vi "PowerGenerated.vi"() -> ()   [LabVIEW 2019]
uses:
  SubVis/Location.ctl
  <vilib>/Analysis/baseanly.llb/Mean (DBL).vi
  <vilib>/Utility/file.llb/Read Delimited Spreadsheet (DBL).vi
  <vilib>/Analysis/NI_AALBase.lvlib
panel:
  out "Day of Max Power":i32 caption="Day:"
  out "Max Power":dbl caption="Max Power:" format="%#_3pW"
  in  "Location":T1
  out "Max Power (watts)":dbl(slide) caption="2.1MW" scale=0.0..40000000.0 scale format="%#_6pW"
  in  "Stop":bool
  in  "USA":bool
  in  "CostaRica":bool
  in  "Brazil":bool
  in  "India":bool
  in  "Australia":bool
  in  "Japan":bool
  in  "SouthAfrica":bool
  in  "Israel":bool
  in  "Germany":bool
  in  "Days of Month":u8(slide)=30 min=1 max=30 step=1 scale=1.0..30.0
  out "USA_Select":u16(ring)
  out "Germany_Select":u16(ring)
  out "Brazil_Select":u16(ring)
  out "Israel_Select":u16(ring)
  out "India_Select":u16(ring)
  out "Japan_Select":u16(ring)
  out "SouthAfrica_Select":u16(ring)
  out "Australia_Select":u16(ring)
  out "CostaRica_Select":u16(ring)
  out "Wind Speed of All Countries":waveform(dbl)[](graph)
  out "Power Per Country":dbl[](graph)
  # "The day of maximum power output for a given location is determined for all days starting from the first day of the month until the selected day. The power output and corresponding day are displayed numerically and the power output is also displayed on a meter."
  # "Choose the location and day of the month that you would like to be displayed on the Power Per Country graph. All data from the first day of the month up until the selected day will be displayed."
  # "All countries wind speed data over 30 days is displayed on this graph."
  # "TO DO:  \nWind plot gets thicker when country is selected.\nTips slide down from above in semitransparent window."
  # "40MW"
  # "MAX POWER:"
  # "Move the mouse over included countried to see a plot of their power generation capabilities.  The windspeed for the selected county is highlighted in the graph at the lower right.  \n\nThe  Max Power can be viewed in the top right indicator and graphically on the meter at the far right.  The peak Day appears as a dotted line.\n\nThe slide control above selects how many days in the month are viewed."
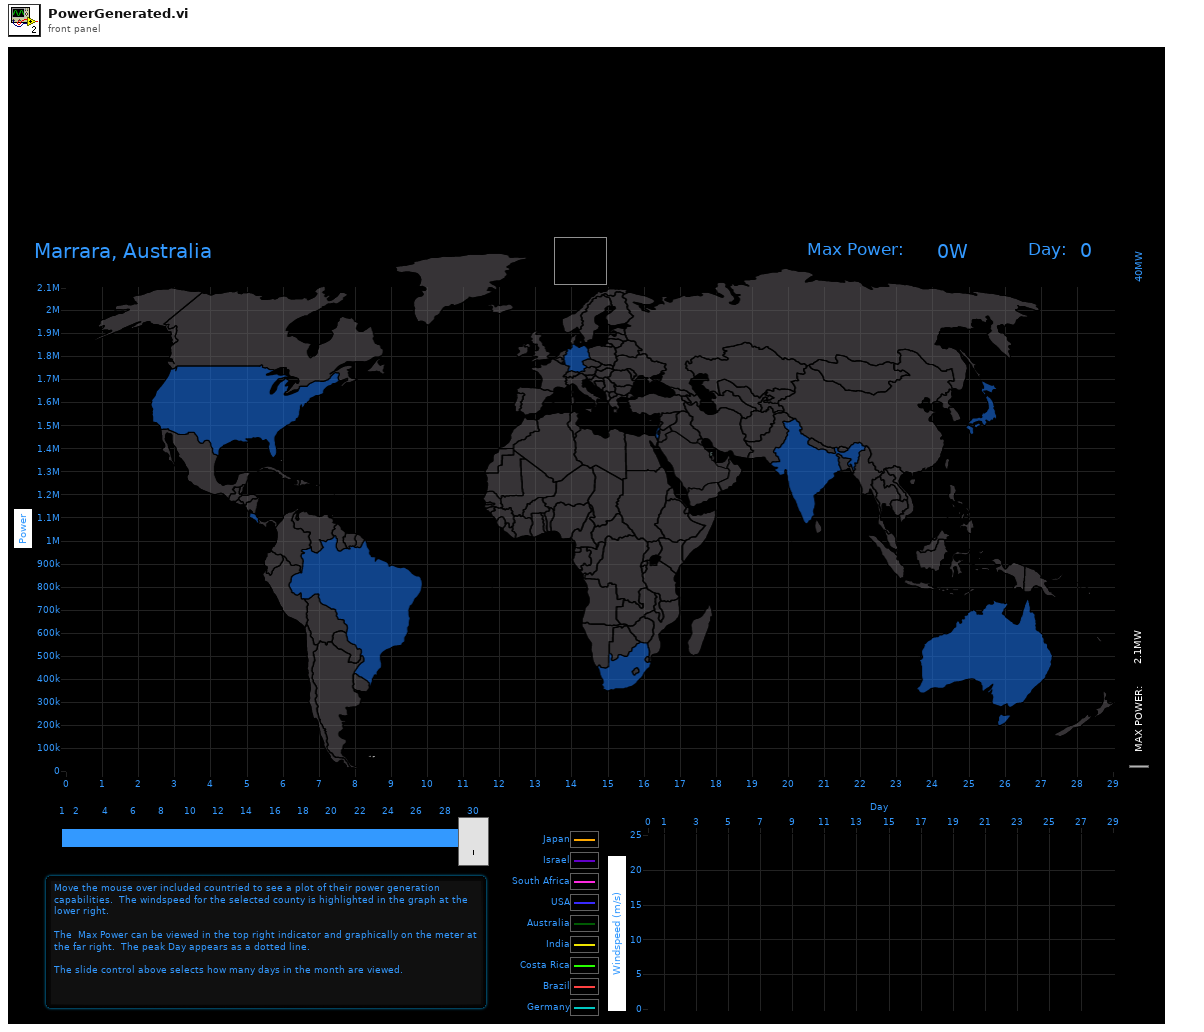
[diagram p1: front panel]
types:
  T1 = typedef "Location.ctl" = enum16{"Marrara, Australia", "Brasilia, Brazil", "Puerto Limon, Costa Rica", "Berlin, Germany", "Mumbai, India", "Sde-Dov, Israel", "Ise Bay, Japan", "Cape Good Hope, South Africa", "Texas, USA"}
  T2 = enum32{"invalid app kind", "Development System", "Run Time System", "Student Edition", "Embedded LabVIEW", "Evaluation", "Custom"}
  T3 = cluster{"Name":string, "Color":u32, "Style":u8, "Point Style":u8, "Name Visible":bool, "Allow Drag":bool, "Cursor Mode":u32, "Plot":i32, "Index":i32, "Position":cluster{"X":i32, "Y":i32}, "X Scale":u32, "Y Scale":u32, "Watch Plots":i32[], "Watch All Plots":bool, "Plot Area":i32, "Label Offset":cluster{"X":dbl, "Y":dbl}}
  T4 = cluster{"Name":string, "Color":u32, "Style":u8, "Point Style":u8, "Name Visible":bool, "Allow Drag":bool, "Annotation Mode":u32, "Plot":i32, "Index":i32, "Position":cluster{"X":dbl, "Y":dbl}, "X Scale":u32, "Y Scale":u32, "Show Arrow":bool, "Lock Name":bool, "Plot Area":i32, "Label Offset":cluster{"X":dbl, "Y":dbl}}
  T5 = cluster{"Location":T1, "Max Power":dbl, "Days of Month":u8, "Power Per Country":dbl[], "Day of Max Power":i32}
  T6 = cluster{"Name":string, "Color":u32, "Style":u8, "Point Style":u8, "Name Visible":bool, "Allow Drag":bool, "Annotation Mode":u32, "Plot":i32, "Index":i32, "Position":cluster{"X":dbl, "Y":dbl}, "X Scale":u32, "Y Scale":u32, "Show Arrow":bool, "Lock Name":bool, "Plot Area":i32, "Label Offset":cluster{"X":dbl, "Y":dbl}}[]
  T7 = cluster{"Name":string, "Color":u32, "Style":u8, "Point Style":u8, "Name Visible":bool, "Allow Drag":bool, "Cursor Mode":u32, "Plot":i32, "Index":i32, "Position":cluster{"X":i32, "Y":i32}, "X Scale":u32, "Y Scale":u32, "Watch Plots":i32[], "Watch All Plots":bool, "Plot Area":i32, "Label Offset":cluster{"X":dbl, "Y":dbl}}[]
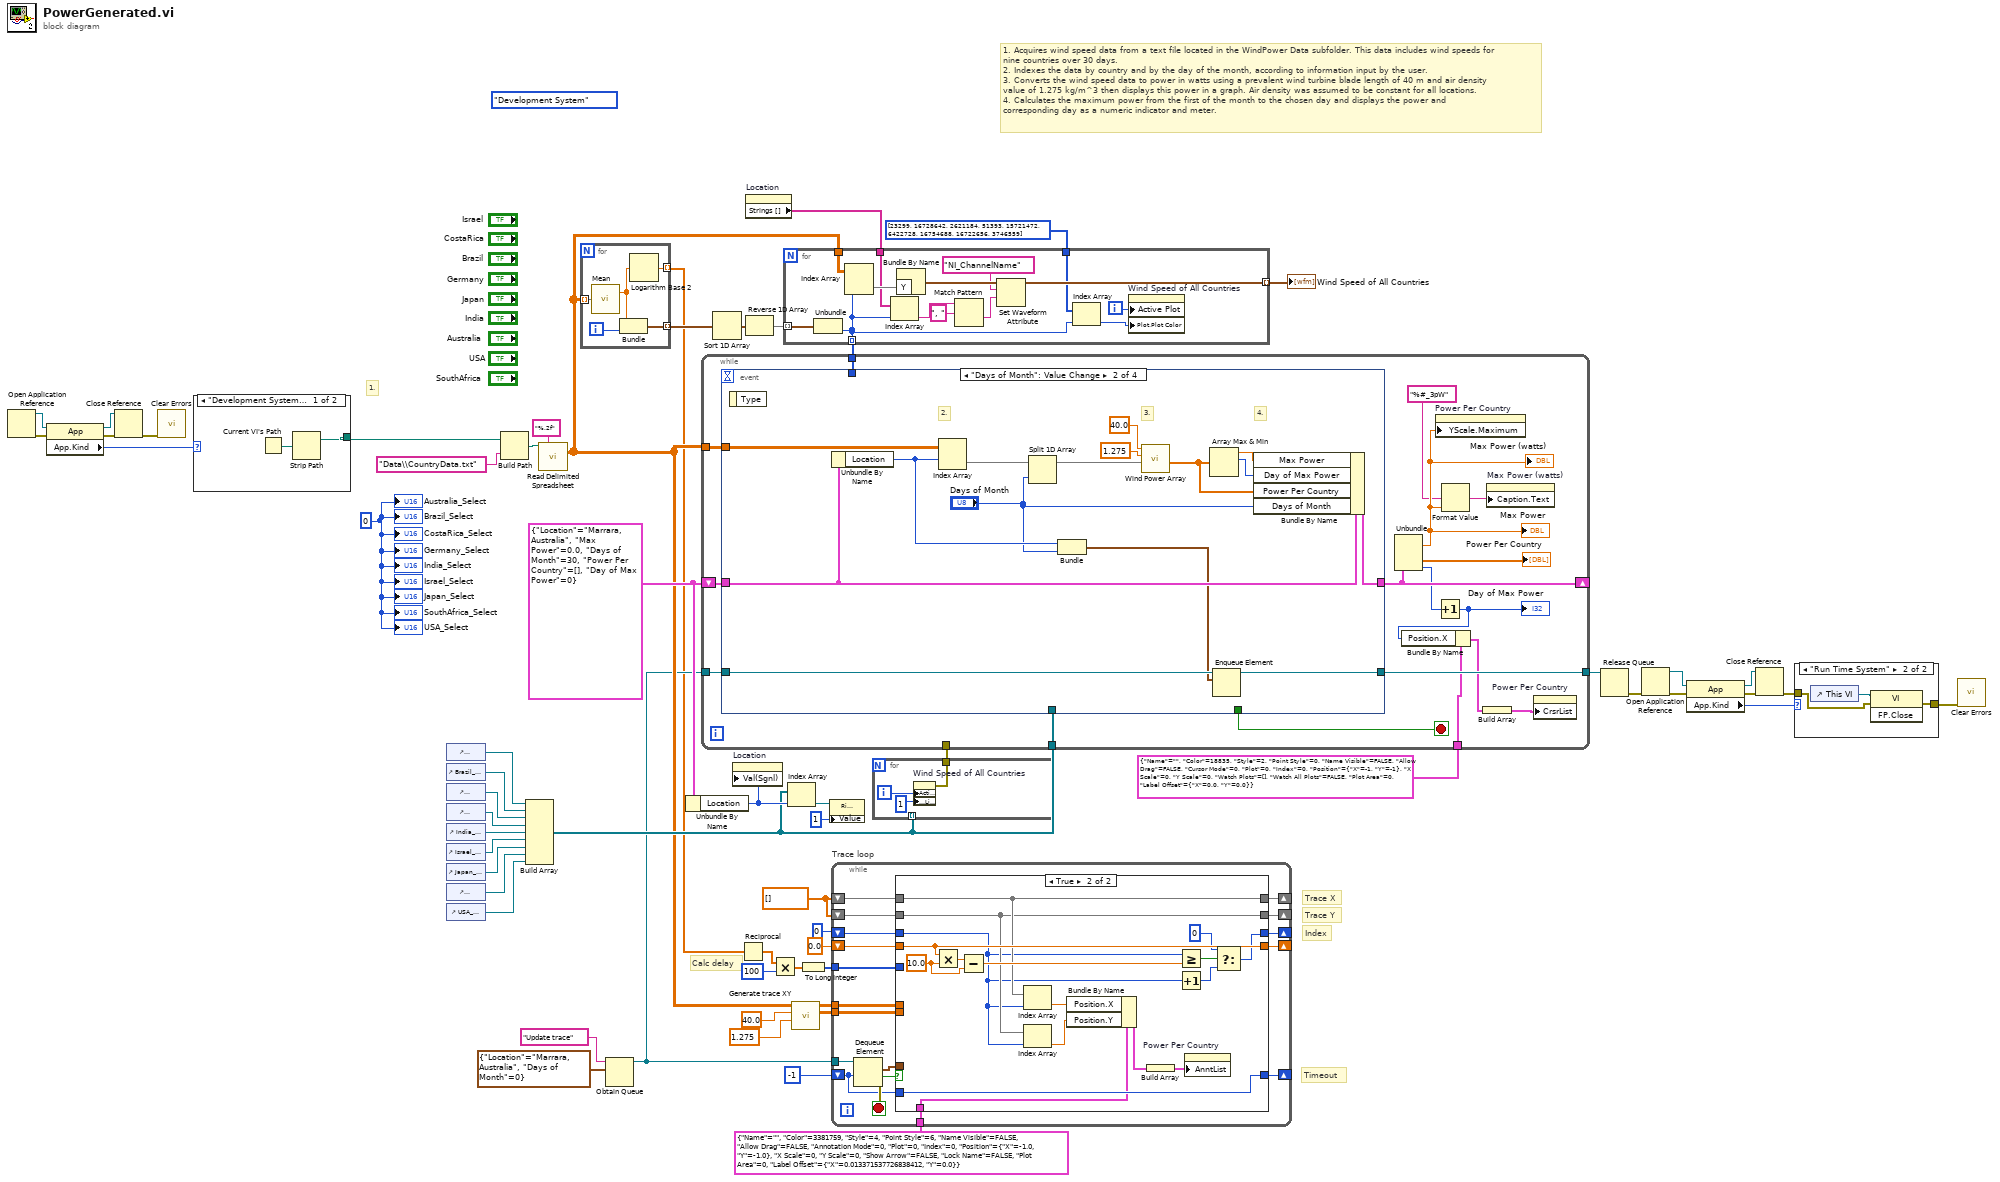
[diagram p0: block diagram]
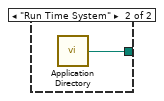
[diagram p3: hidden frame]
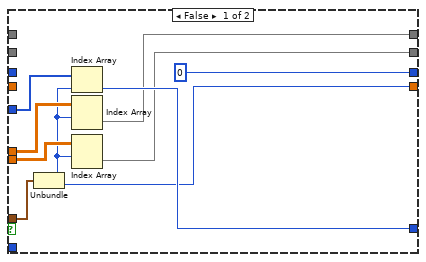
[diagram p4: hidden frame]
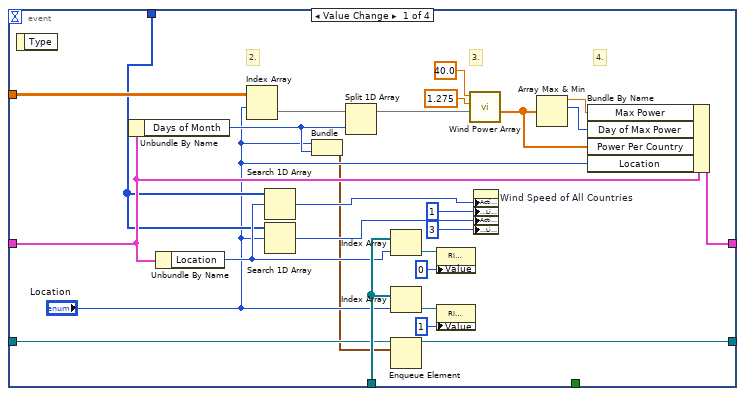
[diagram p5: hidden frame]
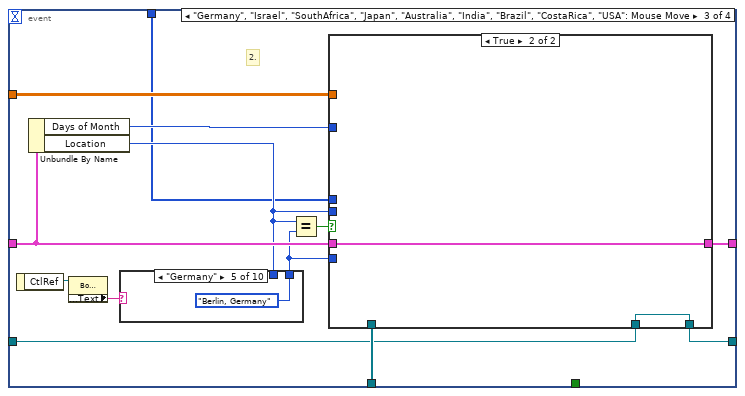
[diagram p6: hidden frame]
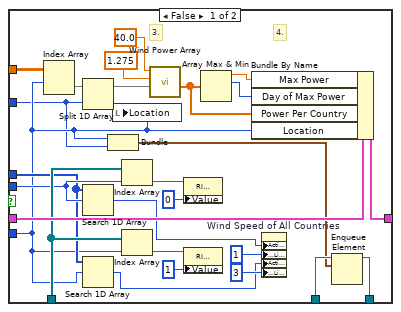
[diagram p7: hidden frame]
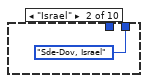
[diagram p9: hidden frame]
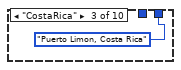
[diagram p10: hidden frame]
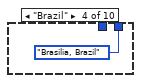
[diagram p11: hidden frame]
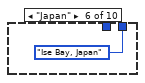
[diagram p12: hidden frame]
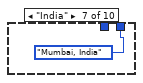
[diagram p13: hidden frame]
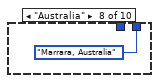
[diagram p14: hidden frame]
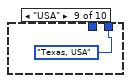
[diagram p15: hidden frame]
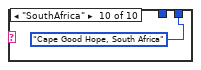
[diagram p16: hidden frame]
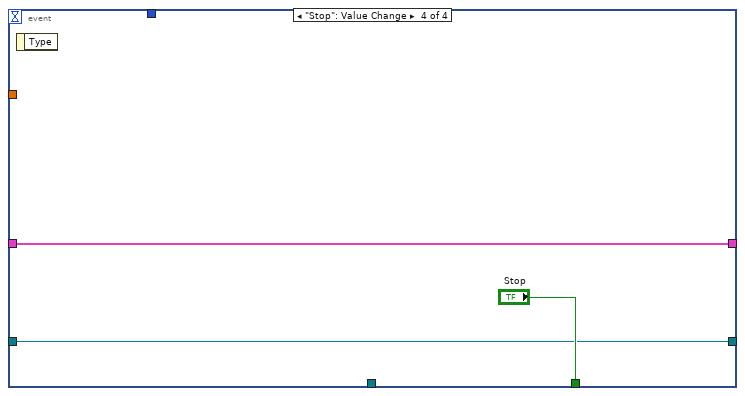
[diagram p17: hidden frame]
diagram:
  (unwired) T2."Development System" ("Application:Kind")
  w25 = dbl[] [] ("Trace X")
  w59 = u16 0 ("Japan_Select")
  w47 = T5 {"Location"=enum."Marrara, Australia", "Max Power"=0.0, "Days of Month"=30, "Power Per Country"=[], "Day of Max Power"=0}
  # "Index"
  # "Timeout"
  # "Trace Y"
  # "Trace X"
  # "Calc delay"
  # "1."
  # "1. Acquires wind speed data from a text file located in the WindPower Data subfolder. This data includes wind speeds for nine countries over 30 days.\n2. Indexes the data by country and by the day of the month, according to information input by the user.\n3. Converts the wind speed data to power in watts using a prevalent wind turbine blade length of 40 m and air density value of 1.275 kg/m^3 then displays this power in a graph. Air density was assumed to be constant for all locations.\n4. Calculates the maximum power from the first of the month to the chosen day and displays the power and corresponding day as a numeric indicator and meter."
  n1 = Open Application Reference() -> (0:w14:errorcluster, 3:w15:refnum<vi>)  [unwired: 4 in]
  n2 = property class="App"(reference=w15, error in=w14) -> (reference out=w12:refnum<vi>, error out=w13:errorcluster, "App.Kind"=w11:T2)
  n3 = Close Reference(reference=w12, error in (no error)=w13) -> (error out=w9:errorcluster)
  n4 = call <vilib>:"Clear Errors.vi"("error in (no error)"=w9) -> ()  [unwired: 5 in, 2 out]
  n5 = case shown="\"Development System\", Default" w11 {
    tunnel: [w62 w64] -> w10
    frame "Development System", Default {
      n6 = Current VI's Path() -> (path=w63:path)
      n7 = Strip Path(path=w63) -> (stripped path=w62:path)  [unwired: 1 out]
    }
    frame "Run Time System" {
      n8 = call <vilib>:"Application Directory.vi"() -> ("Application Directory"=w64:path)
    }
  }
  n9 = control-ref of="Australia_Select"() -> (w58:refnum<vi>)
  n10 = control-ref of="Brazil_Select"() -> (w57:refnum<vi>)
  n11 = control-ref of="CostaRica_Select"() -> (w56:refnum<vi>)
  n12 = control-ref of="Germany_Select"() -> (w55:refnum<vi>)
  n13 = control-ref of="India_Select"() -> (w54:refnum<vi>)
  n14 = control-ref of="Israel_Select"() -> (w53:refnum<vi>)
  n15 = control-ref of="Japan_Select"() -> (w52:refnum<vi>)
  n16 = control-ref of="SouthAfrica_Select"() -> (w51:refnum<vi>)
  n17 = control-ref of="USA_Select"() -> (w50:refnum<vi>)
  n18 = Build Path(base path=w10, name or relative path="Data\\CountryData.txt") -> (appended path=w60:path)
  n19 = Build Array(w58, w57, w56, w55, w54, w53, w52, w51, w50) -> (w38:refnum<vi>[])
  n20 = call-poly <vilib>:"Read Delimited Spreadsheet.vi"("file path (dialog if empty)"=w60, "format (%.3f)"="%.2f") -> ("all rows"=w36:dbl[][])  [unwired: 8 in, 5 out]
  n21 = for {
    tunnel: w36 -> [w69] mode=indexing
    tunnel: [w67] -> w45 mode=indexing
    tunnel: [w65] -> w18 mode=indexing
    i -> [w68]
    n22 = call-poly <vilib>:"Mean.vi"("X"=w69) -> ("mean"=w66:dbl)  [unwired: 1 out]
    n23 = Bundle("mean"=w66, w68) -> (w67:cluster{"mean":dbl, i32})  [unwired: 1 in]
    n24 = Logarithm Base 2(1:w66) -> (0:w65:dbl)
  }
  n25 = Obtain Queue(name (unnamed)="Update trace", element data type=cluster{"Location":T1, "Days of Month":u8} {"Location"=enum."Marrara, Australia", "Days of Month"=0} ("cluster")) -> (queue out=w21:refnum<queue>)  [unwired: 3 in, 2 out]
  n26 = Unbundle By Name(w47) -> ("Location"=w46:T1)
  n27 = Sort 1D Array(array=w45) -> (sorted array=w42:cluster{"mean":dbl, i32}[])
  n28 = property on="Location" class="Enum (strict)"("Val(Sgnl)"=w46) -> ()  [unwired: 2 in, 2 out]
  n29 = Reciprocal(x=w18) -> (1/x=w19:dbl[])
  n30 = property on="Location" class="Enum (strict)"() -> ("Strings []"=w43:string[])  [unwired: 2 in, 2 out]
  n31 = Reverse 1D Array(array=w42) -> (reversed array=w41:cluster{"mean":dbl, i32}[])
  n32 = Multiply(x=w19, y=100 ("Numeric")) -> (x*y=w30:dbl[])
  n33 = for {
    tunnel: w41 -> [w83] mode=indexing
    tunnel: w36 -> [w82]
    tunnel: [w71] -> w40 mode=indexing
    tunnel: [w79] -> w44 mode=indexing
    tunnel: w43 -> [w77]
    tunnel: u32[] [23299, 16728642, 2621184, 51393, 15721472, 6422728, 16754688, 16722656, 3746559] ("Array") -> [w72]
    i -> [w73]
    n34 = Unbundle(w83) -> (w71:i32)  [unwired: 1 out]
    n35 = Index Array(array=w82, index (row)=w71) -> (element=w81:dbl[])  [unwired: 1 in]
    n36 = Index Array(array=w77, index=w71) -> (element=w75:string)
    n37 = Bundle By Name("Y"=w81) -> (w80:waveform(dbl))  [unwired: 1 in]
    n38 = Match Pattern(string=w75, regular expression=", ") -> (after substring=w74:string)  [unwired: 1 in, 3 out]
    n39 = Set Waveform Attribute(5:w74, 6:"NI_ChannelName" ("name"), 7:w80) -> (3:w79:waveform(dbl))  [unwired: 1 in, 2 out]
    n40 = Index Array(array=w72, index=w71) -> (element=w70:u32)
    n41 = property on="Wind Speed of All Countries" class="WFGraph (strict)"("Active Plot"=w73, "Plot.Plot Color"=w70) -> ()  [unwired: 2 in, 2 out]
  }
  "Wind Speed of All Countries" <- w44
  n42 = Index Array(array=w38, index=w46) -> (element=w48:refnum<vi>)
  n43 = call "Generate trace XY.vi"("Density"=1.275, "Blade Lenth"=40.0, "Windspeeds"=w36) -> ("Trace Y"=w27:dbl[][], "Trace X"=w28:dbl[][])  [unwired: 7 in]
  n44 = To Long Integer(number=w30) -> (32bit integer=w29:i32[])
  n45 = property class="Ring (strict)"(reference=w48, "Value"=u16 1) -> ()  [unwired: 1 in, 2 out]
  n46 = while "Trace loop" {
    tunnel: w21 -> [w101]
    tunnel: w29 -> [w95]
    tunnel: w28 -> [w97]
    tunnel: w27 -> [w96]
    shift-right: [w94] -> _
    shift-left: -1 ("timeout in ms (-1)") -> [w89]
    shift-right: [w93] -> _
    shift-left: w25 -> [w92]
    shift-right: [w90] -> _
    shift-left: w25 -> [w91]
    shift-right: [w88] -> _
    shift-left: 0 ("element") -> [w86]
    shift-right: [w87] -> _
    shift-left: 0.0 ("Days of Month") -> [w85]
    tunnel: T4 {"Name"="", "Color"=3381759, "Style"=4, "Point Style"=6, "Name Visible"=FALSE, "Allow Drag"=FALSE, "Annotation Mode"=0, "Plot"=0, "Index"=0, "Position"={"X"=-1.0, "Y"=-1.0}, "X Scale"=0, "Y Scale"=0, "Show Arrow"=FALSE, "Lock Name"=FALSE, "Plot Area"=0, "Label Offset"={"X"=0.013371537726838412, "Y"=0.0}} -> [w84]
    stop <- w100 stop-if-true
    n47 = Dequeue Element(queue=w101, timeout in ms (-1)=w89) -> (element=w98:cluster{"Location":T1, "Days of Month":u8}, timed out?=w99:bool, error out=w100:errorcluster)  [unwired: 1 in, 1 out]
    n48 = case shown="True" w99 {
      tunnel: w98 -> [w111 _]
      tunnel: w97 -> [w109 _]
      tunnel: w96 -> [w110 _]
      tunnel: w95 -> [w107 _]
      tunnel: [w106 w128] -> w94
      tunnel: w89 -> [_ w128]
      tunnel: [w105 w115] -> w93
      tunnel: w92 -> [_ w115]
      tunnel: w91 -> [_ w114]
      tunnel: [w104 w114] -> w90
      tunnel: [0 ("element") w120] -> w88
      tunnel: [w102 w127] -> w87
      tunnel: w86 -> [_ w112]
      tunnel: w85 -> [_ w127]
      tunnel: w84 -> [_ w117]
      frame False {
        n49 = Unbundle(w111) -> ("Location"=w108:T1, "Days of Month"=w102:u8)
        n50 = Index Array(array=w107, index=w108) -> (element=w106:i32)
        n51 = Index Array(array=w109, index (row)=w108) -> (element=w105:dbl[])  [unwired: 1 in]
        n52 = Index Array(array=w110, index (row)=w108) -> (element=w104:dbl[])  [unwired: 1 in]
      }
      frame True {
        w125 = 10.0 ("y")
        n53 = Multiply(x=w127, y=w125) -> (x*y=w126:dbl)
        n54 = Subtract(x=w126, y=w125) -> (x-y=w124:dbl)
        n55 = Index Array(array=w115, index=w112) -> (element=w116:dbl)
        n56 = Index Array(array=w114, index=w112) -> (element=w113:dbl)
        n57 = Bundle By Name(cluster=w117, "Position.X"=w116, "Position.Y"=w113) -> (w118:T4)
        n58 = Build Array(w118) -> (w119:T6)
        n59 = Greater Or Equal?(x=w112, y=w124) -> (x >= y?=w123:bool)
        n60 = Increment(x=w112) -> (x+1=w122:i32)
        n61 = property on="Power Per Country" class="WFGraph (strict)"("AnntList"=w119) -> ()  [unwired: 2 in, 2 out]
        n62 = Select(t=0, s=w123, f=w122) -> (s? t:f=w120:i32)
      }
    }
  }
  n63 = for {
    tunnel: w38 -> [_] mode=indexing
    tunnel: [w129] -> w37
    i -> [w131]
    n64 = property on="Wind Speed of All Countries" class="WFGraph (strict)"("Active Plot"=w131, "Plot.Line Width"=u8 1 ("f")) -> (error out=w129:errorcluster)  [unwired: 2 in, 1 out]
  }
  n65 = while {
    tunnel: w36 -> [w148]
    shift-right: [w145] -> _
    shift-left: w47 -> [w146]
    tunnel: w38 -> [w142]
    tunnel: w40 -> [w141]
    tunnel: w37 -> [_]
    tunnel: w21 -> [w137]
    tunnel: [w136] -> w20
    tunnel: T3 {"Name"="", "Color"=18835, "Style"=2, "Point Style"=0, "Name Visible"=FALSE, "Allow Drag"=FALSE, "Cursor Mode"=0, "Plot"=0, "Index"=0, "Position"={"X"=-1, "Y"=-1}, "X Scale"=0, "Y Scale"=0, "Watch Plots"=[], "Watch All Plots"=FALSE, "Plot Area"=0, "Label Offset"={"X"=0.0, "Y"=0.0}} ("element") -> [w134]
    stop <- w147 stop-if-true
    n66 = event shown="[1] \"Days of Month\": Value Change" {
      selector: _ -> [_ _ _ _]
      dyn-events: _ -> [_ _ _ _]
      timeout: _ -> [_ _ _ _]
      tunnel: w148 -> [w174 w185 w200 _]
      tunnel: [_ _ _ "Stop"] -> w147
      tunnel: w146 -> [w160 w183 w198 w242]
      tunnel: [w166 w184 w197 w242] -> w145
      tunnel: w142 -> [w161 _ w196 _]
      tunnel: w141 -> [w155 _ w192 _]
      tunnel: w137 -> [w151 w179 w191 w241]
      tunnel: [w149 w178 w190 w241] -> w136
      event Value Change {
        # "4."
        # "3."
        # "2."
        n67 = event-data() -> ()  [unwired: 1 in, 1 out]
        n68 = Unbundle By Name(w160) -> ("Days of Month"=w153:u8)
        n69 = Unbundle By Name(w160) -> ("Location"=w157:T1)
        n70 = Index Array "Index Array"(array=w174, index (row)="Location") -> (element=w171:dbl[])  [unwired: 1 in]
        n71 = Search 1D Array(1D array=w155, element=w157) -> (index of element=w156:i32)  [unwired: 1 in]
        n72 = Search 1D Array(1D array=w155, element="Location") -> (index of element=w154:i32)  [unwired: 1 in]
        n73 = Bundle("Location"="Location", "Days of Month"=w153) -> (w150:cluster{"Location":T1, "Days of Month":u8})  [unwired: 1 in]
        n74 = Split 1D Array(array=w171, index=w153) -> (first subarray=w170:dbl[])  [unwired: 1 out]
        n75 = Index Array(array=w161, index=w157) -> (element=w165:refnum<vi>)
        n76 = Index Array(array=w161, index="Location") -> (element=w163:refnum<vi>)
        n77 = Enqueue Element(queue=w151, element=w150) -> (queue out=w149:refnum<queue>)  [unwired: 2 in, 2 out]
        n78 = property class="Ring (strict)"(reference=w165, "Value"=u16 0) -> ()  [unwired: 1 in, 2 out]
        n79 = property class="Ring (strict)"(reference=w163, "Value"=u16 1) -> ()  [unwired: 1 in, 2 out]
        n80 = call "Wind Power Array.vi"("Wind Speed (m/s)"=w170, "Density (kg/m^3)"=1.275 ("Density"), "Blade Length (m)"=40.0 ("Blade Lenth")) -> ("Power (watts)"=w169:dbl[])  [unwired: 8 in]
        n81 = property on="Wind Speed of All Countries" class="WFGraph (strict)"("Active Plot"=w156, "Plot.Line Width"=u8 1, "Active Plot"=w154, "Plot.Line Width"=u8 3) -> ()  [unwired: 2 in, 2 out]
        n82 = Array Max & Min(array=w169) -> (max value=w168:dbl, max index (indices)=w167:i32)  [unwired: 2 out]
        n83 = Bundle By Name(cluster=w160, "Max Power"=w168, "Day of Max Power"=w167, "Power Per Country"=w169, "Location"="Location") -> (w166:T5)
      }
      event "Days of Month": Value Change {
        # "4."
        # "3."
        # "2."
        n84 = event-data() -> ()  [unwired: 1 in, 1 out]
        n85 = Unbundle By Name(w183) -> ("Location"=w177:T1)
        n86 = Index Array "Index Array"(array=w185, index (row)=w177) -> (element=w187:dbl[])  [unwired: 1 in]
        n87 = Split 1D Array(array=w187, index="Days of Month") -> (first subarray=w186:dbl[])  [unwired: 1 out]
        n88 = Bundle("Location"=w177, "Days of Month"="Days of Month") -> (w175:cluster{"Location":T1, "Days of Month":u8})  [unwired: 1 in]
        n89 = call "Wind Power Array.vi"("Wind Speed (m/s)"=w186, "Density (kg/m^3)"=1.275 ("Density"), "Blade Length (m)"=40.0 ("Blade Lenth")) -> ("Power (watts)"=w182:dbl[])  [unwired: 8 in]
        n90 = Array Max & Min(array=w182) -> (max value=w181:dbl, max index (indices)=w180:i32)  [unwired: 2 out]
        n91 = Enqueue Element(queue=w179, element=w175) -> (queue out=w178:refnum<queue>)  [unwired: 2 in, 2 out]
        n92 = Bundle By Name(cluster=w183, "Max Power"=w181, "Day of Max Power"=w180, "Power Per Country"=w182, "Days of Month"="Days of Month") -> (w184:T5)
      }
      event "Germany", "Israel", "SouthAfrica", "Japan", "Australia", "India", "Brazil", "CostaRica", "USA": Mouse Move {
        # "2."
        n93 = event-data() -> ("CtlRef"=w202:refnum<vi>)  [unwired: 1 in]
        n94 = Unbundle By Name(w198) -> ("Days of Month"=w199:u8, "Location"=w195:T1)
        n95 = property class="Bool (strict)"(reference=w202) -> ("Label.Text"=w201:string)  [unwired: 1 in, 2 out]
        n96 = case shown="\"Germany\"" w201 {
          tunnel: [w231 Location."Sde-Dov, Israel" ("Location") Location."Puerto Limon, Costa Rica" ("Location") Location."Brasilia, Brazil" ("Location") Location."Berlin, Germany" ("Location") Location."Ise Bay, Japan" ("Location") Location."Mumbai, India" ("Location") Location."Marrara, Australia" ("Location") Location."Texas, USA" ("Location") Location."Cape Good Hope, South Africa" ("Location")] -> w194
          tunnel: w195 -> [w231 _ _ _ _ _ _ _ _ _]
          frame Default {
          }
          frame "Israel" {
          }
          frame "CostaRica" {
          }
          frame "Brazil" {
          }
          frame "Germany" {
          }
          frame "Japan" {
          }
          frame "India" {
          }
          frame "Australia" {
          }
          frame "USA" {
          }
          frame "SouthAfrica" {
          }
        }
        n97 = Equal?(x=w195, y=w194) -> (x = y?=w193:bool)
        n98 = case shown="True" w193 {
          tunnel: w200 -> [w224 _]
          tunnel: w199 -> [w204 _]
          tunnel: w198 -> [w220 w230]
          tunnel: [w219 w230] -> w197
          tunnel: w196 -> [w218 _]
          tunnel: w195 -> [w209 _]
          tunnel: w194 -> [w205 _]
          tunnel: w192 -> [w208 _]
          tunnel: w191 -> [w207 w229]
          tunnel: [w206 w229] -> w190
          frame False {
            # "4."
            # "3."
            n99 = Index Array(array=w224, index (row)=w205) -> (element=w226:dbl[])  [unwired: 1 in]
            n100 = Split 1D Array(array=w226, index=w204) -> (first subarray=w225:dbl[])  [unwired: 1 out]
            n101 = Search 1D Array(1D array=w208, element=w209) -> (index of element=w211:i32)  [unwired: 1 in]
            n102 = Search 1D Array(1D array=w208, element=w205) -> (index of element=w210:i32)  [unwired: 1 in]
            n103 = Bundle("Location"=w205, "Days of Month"=w204) -> (w203:cluster{"Location":T1, "Days of Month":u8})  [unwired: 1 in]
            n104 = local write "Location"(w205) -> ()
            n105 = Index Array(array=w218, index=w209) -> (element=w217:refnum<vi>)
            n106 = Index Array(array=w218, index=w205) -> (element=w215:refnum<vi>)
            n107 = call "Wind Power Array.vi"("Wind Speed (m/s)"=w225, "Density (kg/m^3)"=1.275 ("Density"), "Blade Length (m)"=40.0 ("Blade Lenth")) -> ("Power (watts)"=w221:dbl[])  [unwired: 8 in]
            n108 = property class="Ring (strict)"(reference=w217, "Value"=u16 0) -> ()  [unwired: 1 in, 2 out]
            n109 = property class="Ring (strict)"(reference=w215, "Value"=u16 1) -> ()  [unwired: 1 in, 2 out]
            n110 = Array Max & Min(array=w221) -> (max value=w222:dbl, max index (indices)=w223:i32)  [unwired: 2 out]
            n111 = Bundle By Name(cluster=w220, "Max Power"=w222, "Day of Max Power"=w223, "Power Per Country"=w221, "Location"=w205) -> (w219:T5)
            n112 = property on="Wind Speed of All Countries" class="WFGraph (strict)"("Active Plot"=w211, "Plot.Line Width"=u8 1, "Active Plot"=w210, "Plot.Line Width"=u8 3) -> ()  [unwired: 2 in, 2 out]
            n113 = Enqueue Element(queue=w207, element=w203) -> (queue out=w206:refnum<queue>)  [unwired: 2 in, 2 out]
          }
          frame True {
          }
        }
      }
      event "Stop": Value Change {
        n114 = event-data() -> ()  [unwired: 1 in, 1 out]
      }
    }
    n115 = Unbundle(w145) -> ("Max Power"=w140:dbl, "Power Per Country"=→"Power Per Country":dbl[], "Day of Max Power"=w143:i32)  [unwired: 2 out]
    "Max Power" <- w140
    "Max Power (watts)" <- w140
    n116 = property on="Power Per Country" class="WFGraph (strict)"("YScale.Maximum"=w140) -> ()  [unwired: 2 in, 2 out]
    n117 = Increment(x=w143) -> (x+1=w133:i32)
    "Day of Max Power" <- w133
    n118 = Bundle By Name(cluster=w134, "Position.X"=w133) -> (w132:T3)
    n119 = Format Value(format string="%#_3pW", value (0)=w140) -> (output string=w138:string)  [unwired: 1 in]
    n120 = Build Array(w132) -> (w135:T7)
    n121 = property on="Max Power (watts)" class="Slide (strict)"("Caption.Text"=w138) -> ()  [unwired: 2 in, 2 out]
    n122 = property on="Power Per Country" class="WFGraph (strict)"("CrsrList"=w135) -> ()  [unwired: 2 in, 2 out]
  }
  n123 = Release Queue(queue=w20) -> (error out=w4:errorcluster)  [unwired: 2 in, 2 out]
  n124 = Open Application Reference(8:w4) -> (0:w7:errorcluster, 3:w8:refnum<vi>)  [unwired: 3 in]
  n125 = property class="App"(reference=w8, error in=w7) -> (reference out=w5:refnum<vi>, error out=w6:errorcluster, "App.Kind"=w3:T2)
  n126 = Close Reference(reference=w5, error in (no error)=w6) -> (error out=w1:errorcluster)
  n127 = case shown="\"Run Time System\"" w3 {
    tunnel: [w244 w247] -> w2
    tunnel: w1 -> [w244 w245]
    frame "Development System", Default {
    }
    frame "Run Time System" {
      n128 = control-ref of="This VI"() -> (w246:refnum<vi>)
      n129 = invoke class="VI" method="FP.Close"(reference=w246, error in=w245) -> (error out=w247:errorcluster)  [unwired: 1 in, 2 out]
    }
  }
  n130 = call <vilib>:"Clear Errors.vi"("error in (no error)"=w2) -> ()  [unwired: 5 in, 2 out]
  "USA_Select" <- w59
  "CostaRica_Select" <- w59
  "Israel_Select" <- w59
  "Germany_Select" <- w59
  "India_Select" <- w59
  "Australia_Select" <- w59
  "Brazil_Select" <- w59
  "Japan_Select" <- w59
  "SouthAfrica_Select" <- w59
